vi "LoadFile.vi"(11 "all rows":string[](array[string])) -> (3 "Array":string[](array[string]))   [LabVIEW 2018]
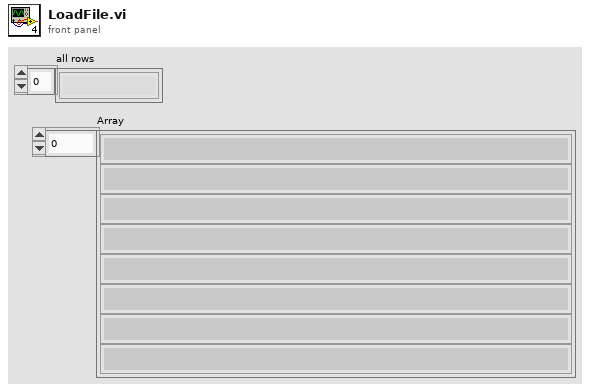
[diagram p1: front panel]
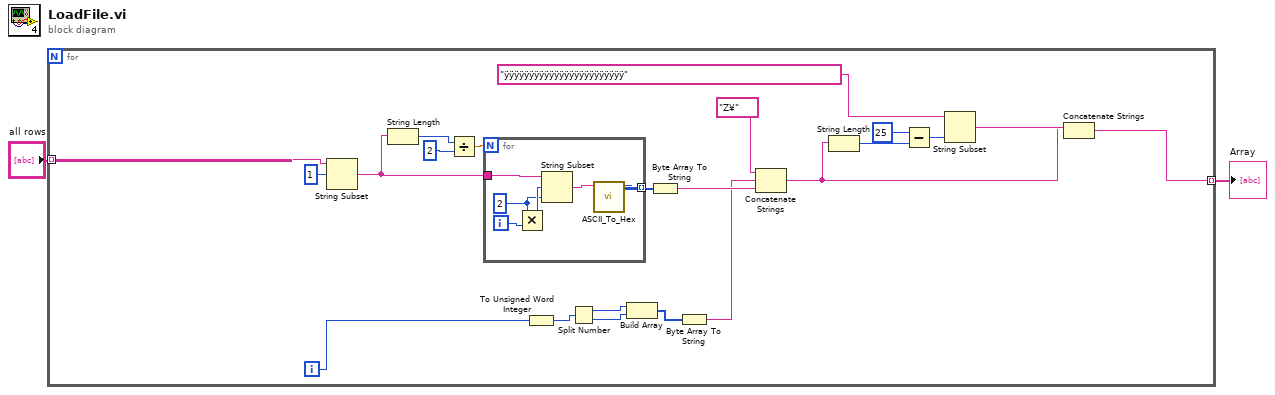
[diagram p0: block diagram]
diagram:
  n1 = for {
    tunnel: "all rows" -> [w18] mode=indexing
    tunnel: [w3] -> w1 mode=indexing
    i -> [w14]
    n2 = String Subset(string=w18, offset (0)=1 ("偏移量(0)")) -> (substring=w19:string)  [unwired: 1 in]
    n3 = String Length(string=w19) -> (length=w23:i32)
    n4 = Divide(x=w23, y=2) -> (x/y=w21:dbl)
    n5 = for {
      N: w21 -> [_]
      tunnel: w19 -> [w30]
      tunnel: [w25] -> w20 mode=indexing
      i -> [w29]
      w27 = 2 ("x")
      n6 = Multiply(x=w27, y=w29) -> (x*y=w28:i32)
      n7 = String Subset(string=w30, offset (0)=w28, length (rest)=w27) -> (substring=w26:string)
      n8 = call "ASCII_To_Hex.vi"("ASCII String"=w26) -> ("hex1"=w25:u8)  [unwired: 6 in, 4 out]
    }
    n9 = To Unsigned Word Integer(number=w14) -> (unsigned 16bit integer=w13:u16)
    n10 = Split Number(x=w13) -> (hi(x)=w12:u8, lo(x)=w11:u8)
    n11 = Build Array(w12, w11) -> (w10:u8[])
    n12 = Byte Array To String(unsigned byte array=w20) -> (string=w17:string)
    n13 = Byte Array To String(unsigned byte array=w10) -> (string=w15:string)
    n14 = Concatenate Strings("Z¥" ("string"), w15, w17) -> (w4:string)
    n15 = String Length(string=w4) -> (length=w9:i32)
    n16 = Subtract(x=25, y=w9) -> (x-y=w6:i32)
    n17 = String Subset(string="ÿÿÿÿÿÿÿÿÿÿÿÿÿÿÿÿÿÿÿÿÿÿÿÿ", length (rest)=w6) -> (substring=w5:string)  [unwired: 1 in]
    n18 = Concatenate Strings(w4, w5) -> (w3:string)
  }
  "Array" <- w1
